vi "DSF.Engine.Plugin.Get Thread ID Pool.vi"(11 "Plugin in":refnum<class "DSF.Engine.Plugin.lvclass">) -> (2 "Thread ID Pool":refnum<class "Pool ID.lvclass">, 3 "Plugin out":refnum<class "DSF.Engine.Plugin.lvclass">)   [LabVIEW 2017, in "Data Sharing Framework Engine.lvlib" / "DSF.Engine.Plugin.lvclass"]
uses:
  DSF.Engine.Plugin.lvclass
  Source/Data Sharing Framework Core/Engine/Execution/Pool/Pool ID/Pool ID.lvclass
  DSF.Engine.Plugin.lvclass/DSF.Engine.Plugin.ctl
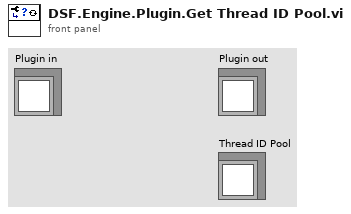
[diagram p1: front panel]
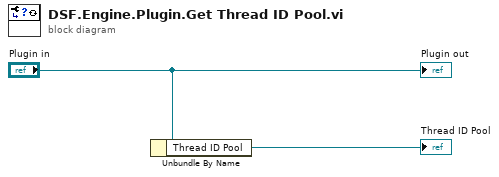
[diagram p0: block diagram]
diagram:
  n1 = Unbundle By Name("Plugin in") -> ("Thread ID Pool"=→"Thread ID Pool":refnum<class "Pool ID.lvclass">)
  "Plugin out" <- "Plugin in"
